vi "test filter.vi"() -> ()   [LabVIEW 2014]
panel:
  in  "Filter type":T1(ring)
  out "Waveform Graph 2":dbl[](graph)
  in  "Avg points":i32
  out "Waveform Graph":dbl[][](graph)
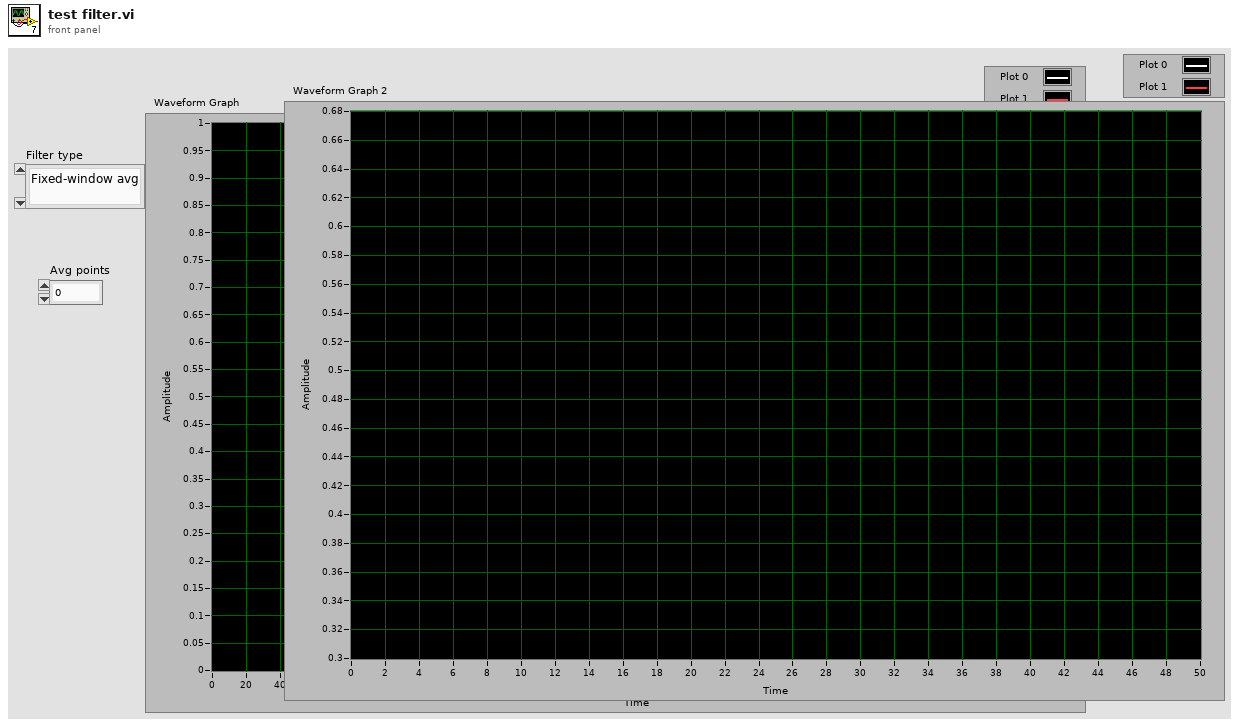
[diagram p1: front panel]
types:
  T1 = enum16{"Fixed-window avg", "Moving-window avg", "F+S-window avg", "S-G filter", "Fixed-window Median", "Moving-window Median "}
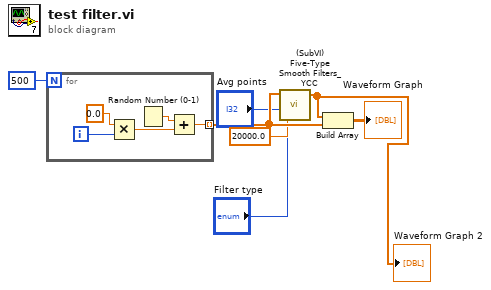
[diagram p0: block diagram]
diagram:
  n1 = for {
    N: 500 -> [_]
    tunnel: [w8] -> w6 mode=indexing
    i -> [w12]
    n2 = Multiply(x=0.0, y=w12) -> (x*y=w10:dbl)
    n3 = Random Number (0-1)() -> (number: 0 to 1=w9:dbl)
    n4 = Add(x=w9, y=w10) -> (x+y=w8:dbl)
  }
  n5 = call "(SubVI) Five-Type Smooth Filters_YCC.vi"("Filter type"="Filter type", "Avg points"="Avg points", "Sampling rate (Hz)"=20000.0, "QPD data"=w6) -> ("Filtered QPD data"=w2:dbl[])  [unwired: 1 in, 1 out]
  "Waveform Graph 2" <- w2
  n6 = Build Array(w2, w6) -> (→"Waveform Graph":dbl[][])
